vi "3D Quadrature (Formula).vi"(8 "tolerance":dbl=1e-05, 9 "Lower Limits":T1, 10 "Upper Limits":T2={"x upper limit"=1.0, "y upper limit"=1.0, "z upper limit"=1.0}, 11 "integrand":string) -> (0 "error":i32, 3 "result":dbl)   [LabVIEW 2020, in "NI_AALPro.lvlib"]
doc: "Performs numerical integration using adaptive quadrature approach. You must manually select the polymorphic instance to use."
uses:
  <vilib>/Analysis/NI_AALPro.lvlib
panel:
  # "Use x,y,z as the independent variables in integrand.\nExample:\nintegrand:  sin(x+y+z)\nx upper = 1, x lower = 0,\ny upper = 1, y lower = 0,\nz upper = 1, z lower = 0,\nresult = 0.879355"
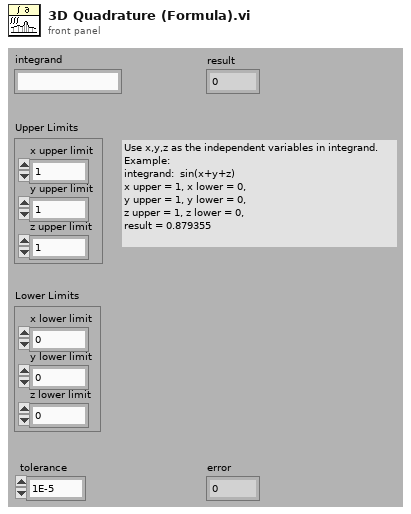
[diagram p1: front panel]
types:
  T1 = cluster{"x lower limit":dbl, "y lower limit":dbl, "z lower limit":dbl}
  T2 = cluster{"x upper limit":dbl, "y upper limit":dbl, "z upper limit":dbl}
  T3 = cluster{"x lower limit":dbl, "x upper limit":dbl}
  T4 = cluster{"y lower limit":dbl, "y upper limit":dbl}
  T5 = cluster{"z lower limit":dbl, "z upper limit":dbl}
  T6 = cluster{cluster{"x lower limit":dbl, "x upper limit":dbl}, cluster{"y lower limit":dbl, "y upper limit":dbl}, cluster{"z lower limit":dbl, "z upper limit":dbl}}
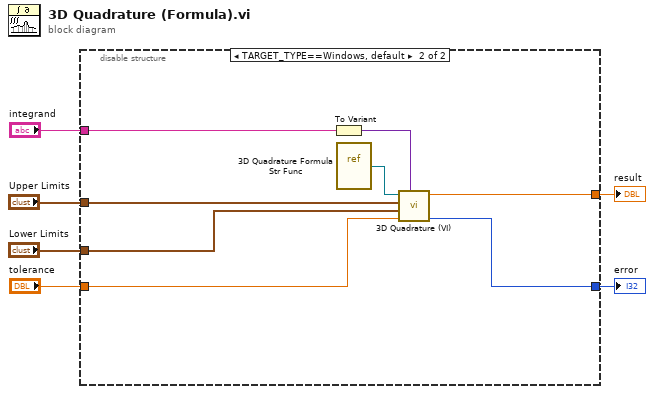
[diagram p0: block diagram]
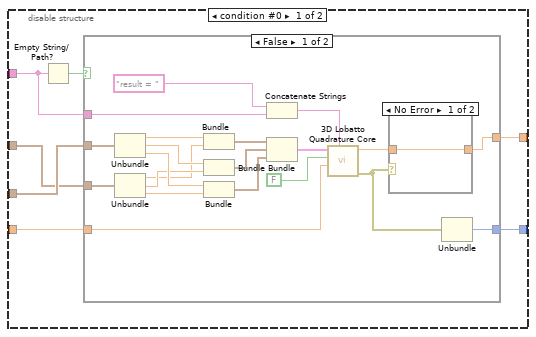
[diagram p2: hidden frame]
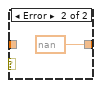
[diagram p3: hidden frame]
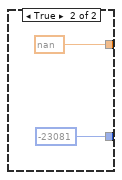
[diagram p4: hidden frame]
diagram:
  n1 = disable-structure shown="TARGET_TYPE==Windows, default" {
    disable-tunnel: [w12 w41] -> w3
    disable-tunnel: "integrand" -> [w11 w43]
    disable-tunnel: "tolerance" -> [w10 w46]
    disable-tunnel: [w9 w45] -> w4
    disable-tunnel: "Upper Limits" -> [w7 w40]
    disable-tunnel: "Lower Limits" -> [w8 w39]
    frame condition #0 {
      n2 = Empty String/Path?(string/path=w11) -> (empty?=w13:bool)
      n3 = case shown="False" w13 {
        tunnel: [w33 nan] -> w9
        tunnel: [w32 -23081] -> w12
        tunnel: w11 -> [w31 _]
        tunnel: w8 -> [w19 _]
        tunnel: w10 -> [w15 _]
        tunnel: w7 -> [w18 _]
        frame False {
          n4 = Unbundle(w19) -> ("x lower limit"=w20:dbl, "y lower limit"=w22:dbl, "z lower limit"=w24:dbl)
          n5 = Unbundle(w18) -> ("x upper limit"=w21:dbl, "y upper limit"=w23:dbl, "z upper limit"=w25:dbl)
          n6 = Bundle("x lower limit"=w20, "x upper limit"=w21) -> (w26:T3)  [unwired: 1 in]
          n7 = Bundle("y lower limit"=w22, "y upper limit"=w23) -> (w27:T4)  [unwired: 1 in]
          n8 = Bundle("z lower limit"=w24, "z upper limit"=w25) -> (w28:T5)  [unwired: 1 in]
          n9 = Concatenate Strings("result = ", w31) -> (w17:string)
          n10 = Bundle(w26, w27, w28) -> (w16:T6)  [unwired: 1 in]
          n11 = call <vilib>:"3D Lobatto Quadrature Core.vi"("formula"=w17, "tolerance"=w15, "Formula/VI ref"=FALSE, "limits"=w16) -> ("error out"=w29:errorcluster, "result"=w34:dbl)  [unwired: 6 in]
          n12 = case shown="No Error" w29 {
            tunnel: w34 -> [w35 _]
            tunnel: [w35 nan] -> w33
            frame No Error {
            }
            frame Error {
            }
          }
          n13 = Unbundle(w29) -> ("code"=w32:i32)  [unwired: 2 out]
        }
        frame True {
        }
      }
    }
    frame condition #1 (active) {
      n14 = To Variant(anything=w43) -> (Variant=w44:variant)
      n15 = vi-ref <vilib>:"3D Quadrature Formula Str Func.vi"() -> (w42:refnum<vi>)
      n16 = call <vilib>:"3D Quadrature (VI).vi"("data"=w44, "tolerance"=w46, "Lower Limits"=w39, "Upper Limits"=w40, "integrand"=w42) -> ("error"=w41:i32, "result"=w45:dbl)  [unwired: 5 out]
    }
  }
  "error" <- w3
  "result" <- w4
